vi "filter data.vi"(6 "graph only (f)":bool, 8 "error in (no error)":errorcluster, 10 "selection filter":T1={"Volume Type"={"Ongoing"=TRUE, "Limited Series"=TRUE, "Annuals"=TRUE, "One Shots"=TRUE, "Reference/Reprints"=TRUE, "Digital"=TRUE}, "team"=[], "characters"=[], "storyArcs"=[], "Plot End"=timestamp(0 s since 1904-01-01), "Plot Start"=timestamp(0 s since 1904-01-01), "title"=[], "colors"={"ongoing"=0, "Limited Series"=0, "Annuals"=0, "One Shots"=0, "Reprints"=0, "Digital"=0}, "concept"=[], "show all"=FALSE, "Search by Title"=enum."AND", "pub ids"=[]}, 11 "manager_daemon in":refnum<class "manager_daemon.lvclass">) -> (0 "error out":errorcluster, 3 "manager_daemon out":refnum<class "manager_daemon.lvclass">)   [LabVIEW 2024, in "manager_daemon.lvclass"]
uses:
  manager_daemon.lvclass
  TypeDefs/graphic.filter--cluster.ctl
  Graphic_UI/typedefs/volume.type.colors--cluster.ctl
  type_defs/msg--cluster.ctl
  type_defs/cmd--enum.ctl
  CV_Shared_Library/CV_Shared_Library.lvlib
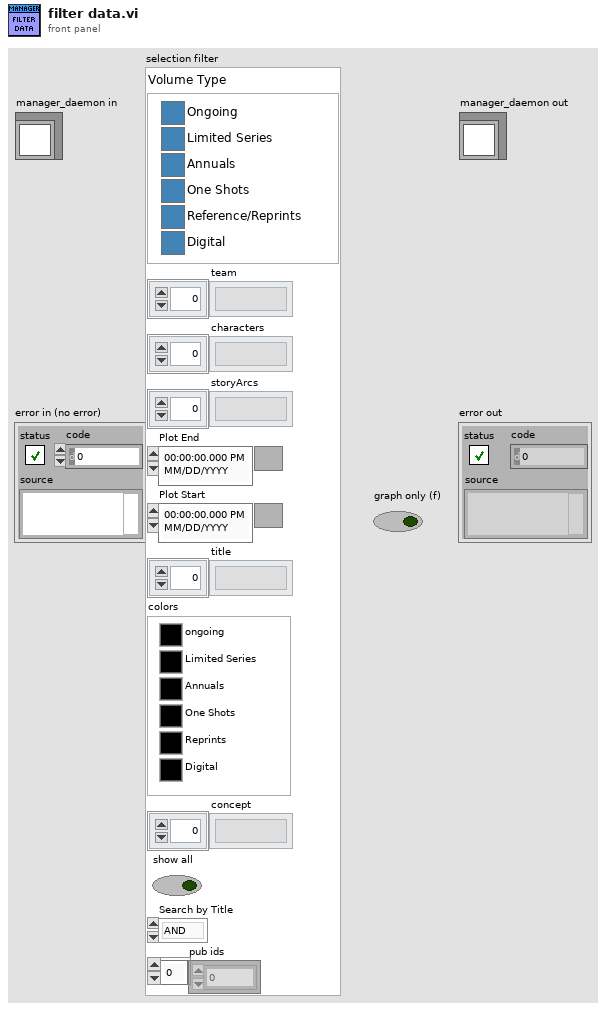
[diagram p1: front panel]
types:
  T1 = typedef "CV_Shared_Library.lvlib/graphic.filter--cluster.ctl" = cluster{"Volume Type":cluster{"Ongoing":bool, "Limited Series":bool, "Annuals":bool, "One Shots":bool, "Reference/Reprints":bool, "Digital":bool}, "team":string[], "characters":string[], "storyArcs":string[], "Plot End":timestamp, "Plot Start":timestamp, "title":string[], "colors":T2, "concept":string[], "show all":bool, "Search by Title":enum32{"AND", "OR"}, "pub ids":i32[]}
  T2 = typedef "volume.type.colors--cluster.ctl" = cluster{"ongoing":u32, "Limited Series":u32, "Annuals":u32, "One Shots":u32, "Reprints":u32, "Digital":u32}
  T3 = typedef "manager_daemon.lvclass/cmd--enum.ctl" = enum16{"init", "run", "load binaries", "save binaries", "updated volume", "get set names", "return vol path by id", "return vol ids by publisher", "display info", "filter release week", "apply filter", "add publisher", "get publishers", "add volume", "add volumes", "add issues", "add issue", "delete volume", "delete issues", "download issues", "scan for reprints", "exit"}
  T4 = typedef "manager_daemon.lvclass/msg--cluster.ctl" = cluster{"cmd":T3, "data":variant}
  T5 = cluster{"selection filter":T1, "graph only (f)":bool}
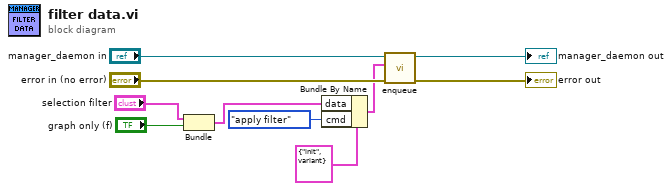
[diagram p0: block diagram]
diagram:
  n1 = Bundle("selection filter"="selection filter", "graph only (f)"="graph only (f)") -> (w1:T5)  [unwired: 1 in]
  n2 = Bundle By Name(cluster=T4 {"cmd"=enum."init", "data"=variant} ("msg"), "data"=w1, "cmd"=cmd--enum."apply filter") -> (w4:T4)
  n3 = call "enqueue.vi"("error in (no error)"="error in (no error)", "msg"=w4, "manager_daemon in"="manager_daemon in") -> ("error out"=→"error out":errorcluster, "manager_daemon out"=→"manager_daemon out":refnum<class "manager_daemon.lvclass">)  [unwired: 7 in]
